vi "SetIndividualJointVelocity.vi"(0 "error in":errorcluster, 2 "Joint States":T1(array[cluster]), 3 "node":string) -> (1 "error out":errorcluster)   [LabVIEW 2012]
doc: "Set individual joint speeds on Baxter"
uses:
  ROS/Code/SubVIs/JointMode.ctl
panel:
  # "Joint Names:\nhead_pan, head_nod\nleft_e1, left e_0, left s_0, left s_1, left w_0, left w_1\nright e_1, right e_0, right s_0, right s_1, right w_0, right w_1"
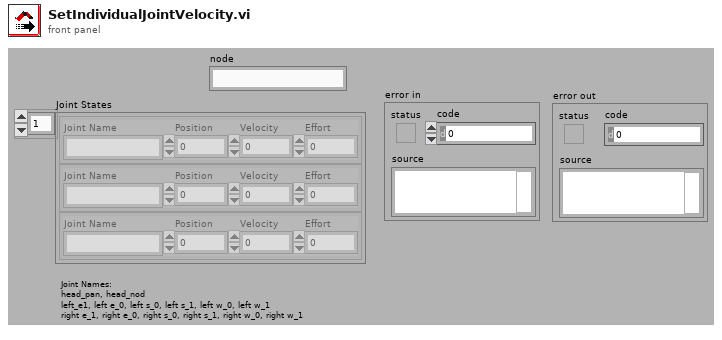
[diagram p1: front panel]
types:
  T1 = cluster{"Joint Name":string, "Position":dbl, "Velocity":dbl, "Effort":dbl}[]
  T2 = typedef "JointMode.ctl" = u8
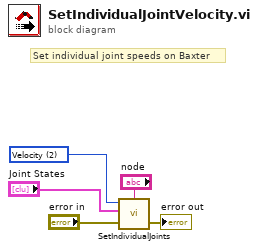
[diagram p0: block diagram]
diagram:
  w4 = T2 2 items=["Position"=1, "Velocity"=2, "Effort"=3] ("Mode")
  # "Set individual joint speeds on Baxter"
  n1 = call "SetIndividualJoints.vi"("node"="node", "Mode"=w4, "Joint States"="Joint States", "error in"="error in") -> ("error out"=→"error out":errorcluster)  [unwired: 2 in]
